vi "Actor Core.vi"(8 "error in":errorcluster, 11 "BuildWorker in":refnum<class "BuildWorker.lvclass">) -> (0 "error out":errorcluster, 3 "Actor out":refnum<class "Actor.lvclass">)   [LabVIEW 2017, in "BuildWorker.lvlib" / "BuildWorker.lvclass"]
doc: "(<B>Filename</B>: Actor Framework.lvlib:Actor.lvclass:Actor Core.vi)\n\nReceives messages to the actor, reacts to them, and initiates any error handling that may shut the actor down.\n\nDescendant classes may override this VI to append parallel tasks for the actor to complete while it handles messages. Overrides use the Call Parent Method node."
uses:
  BuildWorker.lvclass
  C:/Users/Public/Documents/wc/BuildFarm/src/LabVIEW/vi.lib/BenjaminR/Build Farm/Actors/Framework/Actor wUI/Actor wUI.lvclass
  <vilib>/ActorFramework/Actor/Actor.lvclass
  BuildWorker.lvclass/BuildWorker.ctl
  Framework/Actor wUI/Actor wUI.lvclass/Actor wUI.ctl
  Framework/Actor wUI/Write UI Ref.vi
  Framework/Actor wUI/Actor wUI.lvclass
panel:
  out "BuildWorker Name":string
  out "BuildServer Port":u16
  out "context":string
  in  "TaskList":i32(listbox)
  out "status":string
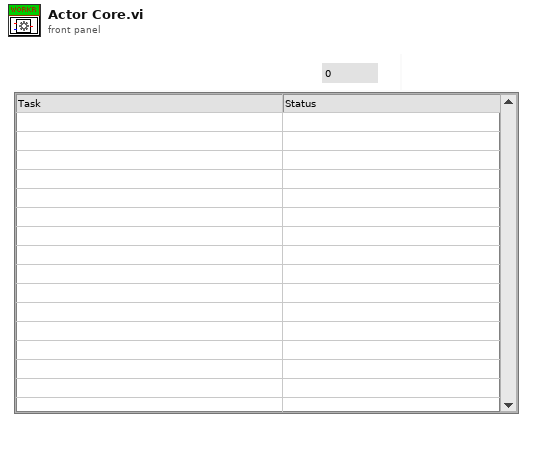
[diagram p1: front panel]
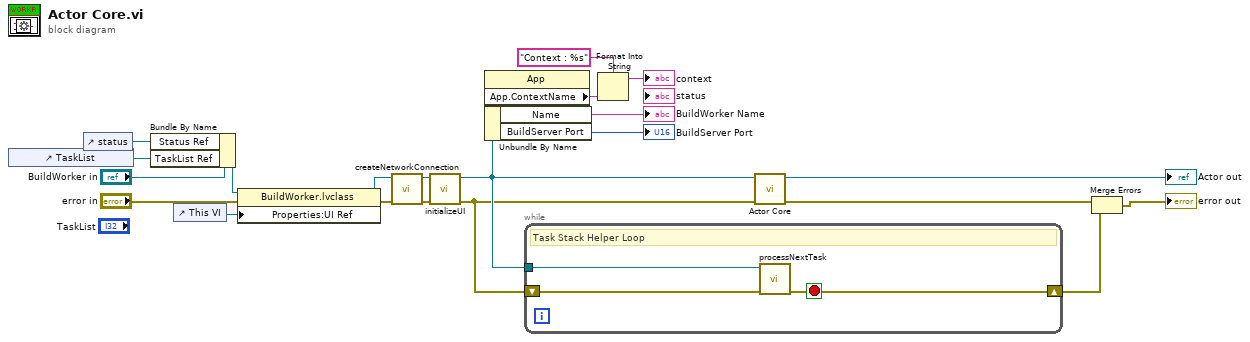
[diagram p0: block diagram]
diagram:
  n1 = control-ref of="TaskList"() -> (w16:refnum<vi>)
  n2 = control-ref of="status"() -> (w12:refnum<vi>)
  n3 = Bundle By Name(cluster="BuildWorker in", "Status Ref"=w12, "TaskList Ref"=w16) -> (w5:refnum<class "BuildWorker.lvclass">)
  n4 = control-ref of="This VI"() -> (w8:refnum<vi>)
  n5 = property class="BuildWorker.lvclass"(reference=w5, error in="error in", "Properties:UI Ref"=w8) -> (reference out=w11:refnum<class "BuildWorker.lvclass">, error out=w9:errorcluster)
  n6 = call "createNetworkConnection.vi"("error in (no error)"=w9, "BuildWorker in"=w11) -> ("error out"=w14:errorcluster, "BuildWorker out"=w7:refnum<class "BuildWorker.lvclass">)  [unwired: 8 in]
  n7 = call "initializeUI.vi"("error in (no error)"=w14, "BuildWorker in"=w7) -> ("error out"=w13:errorcluster, "BuildWorker out"=w15:refnum<class "BuildWorker.lvclass">)  [unwired: 8 in]
  n8 = property class="App"() -> ("App.ContextName"=w3:string)  [unwired: 2 in, 2 out]
  n9 = Unbundle By Name(w15) -> ("Name"=→"BuildWorker Name":string, "BuildServer Port"=→"BuildServer Port":u16)
  n10 = while {
    tunnel: w15 -> [w24]
    shift-right: [w22] -> w18
    shift-left: w13 -> [w23]
    stop <- w22 stop-if-true
    # "Task Stack Helper Loop"
    n11 = call "processNextTask.vi"("error in (no error)"=w23, "BuildWorker in"=w24) -> ("error out"=w22:errorcluster)  [unwired: 8 in, 1 out]
  }
  n12 = Format Into String(format string="Context : %s", w3) -> (resulting string=→"context":string)  [unwired: 2 in, 1 out]
  n13 = call-parent "Actor Core.vi"("error in"=w13, "Actor in"=w15) -> ("error out"=w21:errorcluster, "Actor out"=→"Actor out":refnum<class "Actor.lvclass">)  [unwired: 8 in]
  n14 = Merge Errors(w21, w18) -> (→"error out":errorcluster)
